vi "Pre Launch Init.vi"(11 "SineModel In":refnum<class "SineModel.lvclass">) -> (0 "error out":errorcluster, 3 "SineModel Out":refnum<class "SineModel.lvclass">)   [LabVIEW 2017, in "Dynamic Viewables.lvlib" / "SineModel.lvlib" / "SineModel.lvclass"]
doc: "(<B>Filename</B>: Actor Framework.lvlib:Actor.lvclass:Pre Launch Init.vi)\n\nDefines behavior that occurs after the Launch Nested Actor method is invoked but before the actor's Actor Core method begins running.\n\nBy default, this method does nothing. A descendant class may override it to define behavior.MVA Framework 1.7.0.33\nEthan Stern - Composed Systems\nCopyright (c) 2018, Composed Systems"
uses:
  SineModel.lvclass
  D:/OneDrive/Composed Systems/mva-core/Source/IModel/IModel/IModel.lvclass
  C:/Program Files/National Instruments/LabVIEW 2017/vi.lib/ActorFramework/Actor/Actor.lvclass
  mva-core/Source/IObserver/IObserver/IObserver.lvclass/IObserver.ctl
  mva-core/Source/IModel/IModel/IModel.lvclass/IModel.ctl
  mva-core/Source/IMediator/PublishRequest/PublishRequest.lvclass/PublishRequest.ctl
  mva-core/Source/IMediator/IMediator Messages/Publish Msg/Publish Msg.lvclass/Publish Msg.ctl
  actor-framework-messages/Source/RoundTripMessage/RoundTripMessage.lvclass/RoundTripMessage.ctl
  <vilib>/ActorFramework/Message Enqueuer/Message Enqueuer.lvclass/Message Enqueuer.ctl
  <vilib>/ActorFramework/Actor/Actor.lvclass/Actor.ctl
  <vilib>/ActorFramework/Message Enqueuer/Init from Existing Queue.vi
  <vilib>/ActorFramework/Message Enqueuer/Enqueue.vi
  mva-core/Source/IMediator/IMediator Messages/Publish Msg/Send Pre-Addressed Publish.vi
  mva-core/Source/IObserver/IObserver/Read Unique ID.vi
  mva-core/Source/IMediator/PublishRequest/Pack Publish Request.vi
  actor-framework-messages/Source/RoundTripMessage/Return Round-Trip Message.vi
  mva-core/Source/IModel/IModel/IModel.lvclass
  D:/OneDrive/Composed Systems/mva-core/Source/IObserver/IObserver/IObserver.lvclass
  mva-core/Source/IMediator/IMediator Messages/Publish Msg/Publish Msg.lvclass
  D:/OneDrive/Composed Systems/actor-framework-messages/Source/RoundTripMessage/RoundTripMessage.lvclass
  actor-framework-messages/Source/RoundTripMessage/RoundTripMessage.lvclass
  C:/Program Files/National Instruments/LabVIEW 2017/vi.lib/ActorFramework/Message/Message.lvclass
  SineModel Messages/GenerateSineWave Msg/GenerateSineWave Msg.lvclass
  <vilib>/ActorFramework/Message Priority Queue/Priority Enqueue.vi
  <vilib>/ActorFramework/Message Enqueuer/Message Enqueuer.lvclass
  mva-core/Source/IMediator/PublishRequest/PublishRequest.lvclass
  <vilib>/ActorFramework/Actor/Actor.lvclass
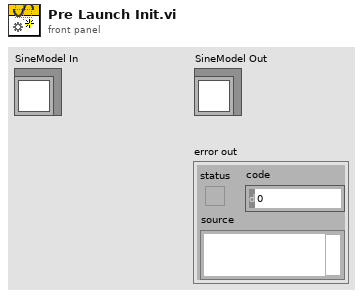
[diagram p1: front panel]
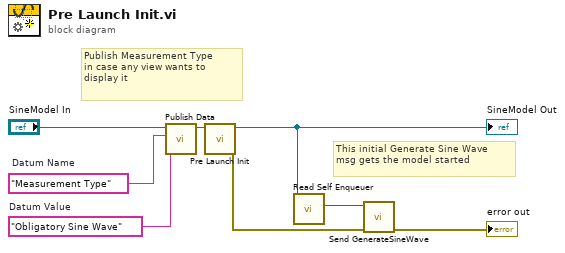
[diagram p0: block diagram]
diagram:
  w1 = "Obligatory Sine Wave"  # Datum Value
  w2 = "Measurement Type"  # Datum Name
  # "Publish Measurement Type\nin case any view wants to\ndisplay it"
  # "This initial Generate Sine Wave\nmsg gets the model started"
  n1 = call "Publish Data.vi"("Data to Publish"=w1, "Datum Name"=w2, "IModel in"="SineModel In") -> ("IModel out"=w3:refnum<class "SineModel.lvclass">)  [unwired: 7 in, 1 out]
  n2 = call-parent "Pre Launch Init.vi"("IModel in"=w3) -> ("error out"=w5:errorcluster, "IModel out"=w7:refnum<class "SineModel.lvclass">)  [unwired: 9 in]
  "SineModel Out" <- w7
  n3 = call <vilib>:"Read Self Enqueuer.vi"("Actor"=w7) -> ("Self Enqueuer"=w6:refnum<class "Message Enqueuer.lvclass">)  [unwired: 10 in]
  n4 = call "Send GenerateSineWave.vi"("error in (no error)"=w5, "Message Enqueuer"=w6) -> ("error out"=→"error out":errorcluster)  [unwired: 8 in, 1 out]
